vi "peak_detection.vi"(0 "Array":dbl[](array[numeric])) -> (1 "upper":dbl[](array[numeric]), 2 "upper time":dbl[](array[numeric]), 3 "lower":dbl[](array[numeric]), 4 "lower time":dbl[](array[numeric]))   [LabVIEW 2018]
panel:
  # "after interplotation"
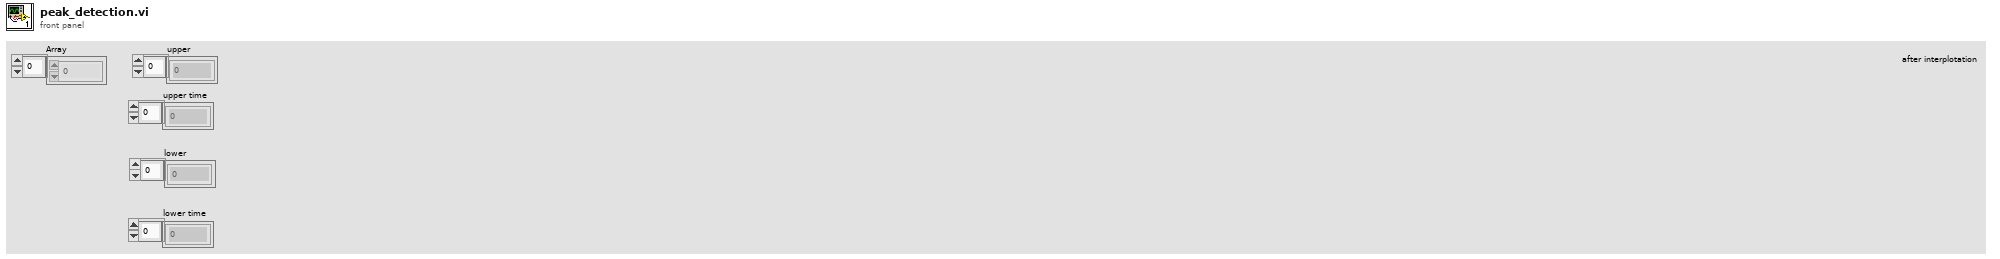
[diagram p1: front panel]
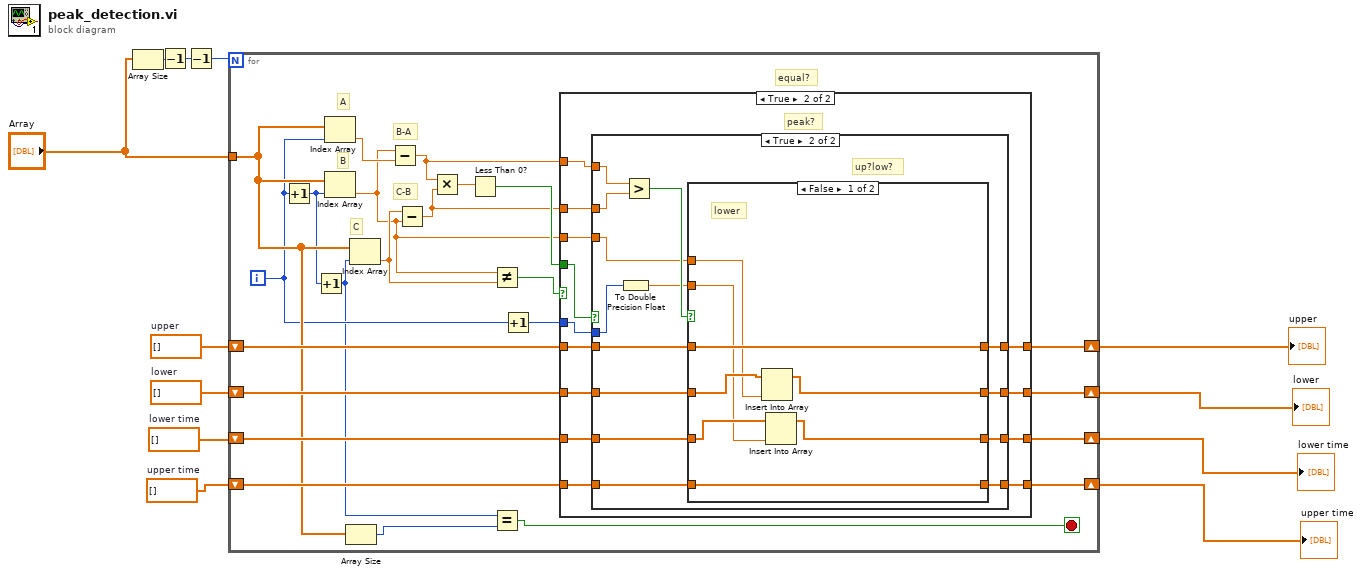
[diagram p0: block diagram]
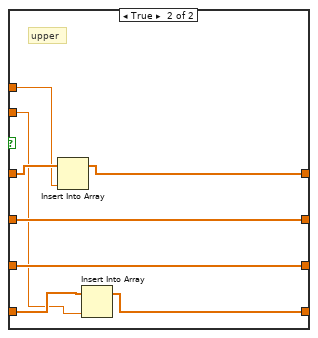
[diagram p4: hidden frame]
diagram:
  w6 = dbl[] []  # upper time
  w5 = dbl[] []  # lower time
  w4 = dbl[] []  # lower
  w3 = dbl[] []  # upper
  n1 = Array Size(array="Array") -> (size(s)=w11:i32)
  n2 = Decrement(x=w11) -> (x-1=w12:i32)
  n3 = Decrement(x=w12) -> (x-1=w1:i32)
  n4 = for {
    N: w1 -> [_]
    tunnel: "Array" -> [w25]
    shift-right: [w30] -> w7
    shift-left: w3 -> [w35]
    shift-right: [w29] -> w8
    shift-left: w4 -> [w34]
    shift-right: [w28] -> w9
    shift-left: w5 -> [w32]
    shift-right: [w27] -> w10
    shift-left: w6 -> [w31]
    i -> [w22]
    stop <- w24 stop-if-true
    # "equal?"
    # "C"
    # "B"
    # "A"
    # "C-B"
    # "B-A"
    n5 = Increment(x=w22) -> (x+1=w23:i32)
    n6 = Increment(x=w23) -> (x+1=w21:i32)
    n7 = Index Array(array=w25, index=w22) -> (element=w20:dbl)
    n8 = Index Array(array=w25, index=w23) -> (element=w13:dbl)
    n9 = Array Size(array=w25) -> (size(s)=w26:i32)
    n10 = Index Array(array=w25, index=w21) -> (element=w16:dbl)
    n11 = Subtract(x=w13, y=w20) -> (x-y=w15:dbl)
    n12 = Subtract(x=w16, y=w13) -> (x-y=w14:dbl)
    n13 = Multiply(x=w15, y=w14) -> (x*y=w19:dbl)
    n14 = Less Than 0?(x=w19) -> (x < 0?=w18:bool)
    n15 = Not Equal?(x=w13, y=w16) -> (x != y?=w17:bool)
    n16 = Equal?(x=w21, y=w26) -> (x = y?=w24:bool)
    n17 = Increment(x=w22) -> (x+1=w33:i32)
    n18 = case shown="True" w17 {
      tunnel: w35 -> [w39 w50]
      tunnel: w33 -> [_ w43]
      tunnel: w34 -> [w38 w48]
      tunnel: w32 -> [w37 w46]
      tunnel: w31 -> [w36 w44]
      tunnel: [w39 w51] -> w30
      tunnel: [w38 w49] -> w29
      tunnel: [w37 w47] -> w28
      tunnel: [w36 w45] -> w27
      tunnel: w18 -> [_ w52]
      tunnel: w15 -> [_ w42]
      tunnel: w14 -> [_ w41]
      tunnel: w13 -> [_ w40]
      frame False {
      }
      frame True {
        # "peak?"
        n19 = case shown="True" w52 {
          tunnel: [w56 w61] -> w51
          tunnel: w50 -> [w56 w62]
          tunnel: [w55 w67] -> w49
          tunnel: w48 -> [w55 w66]
          tunnel: [w54 w65] -> w47
          tunnel: w46 -> [w54 w64]
          tunnel: [w53 w59] -> w45
          tunnel: w44 -> [w53 w60]
          tunnel: w43 -> [_ w58]
          tunnel: w42 -> [_ w70]
          tunnel: w41 -> [_ w69]
          tunnel: w40 -> [_ w63]
          frame False {
          }
          frame True {
            # "up?low?"
            n20 = To Double Precision Float(number=w58) -> (double precision float=w57:dbl)
            n21 = Greater?(x=w70, y=w69) -> (0:w68:bool)
            n22 = case shown="False" w68 {
              tunnel: [w74 w86] -> w67
              tunnel: w66 -> [w76 w86]
              tunnel: [w71 w85] -> w65
              tunnel: w64 -> [w73 w85]
              tunnel: w63 -> [w75 w83]
              tunnel: w62 -> [w78 w84]
              tunnel: [w78 w82] -> w61
              tunnel: w60 -> [w77 w81]
              tunnel: [w77 w79] -> w59
              tunnel: w57 -> [w72 w80]
              frame False {
                # "lower"
                n23 = Insert Into Array(array=w76, new element=w75) -> (w74:dbl[])  [unwired: 1 in]
                n24 = Insert Into Array(array=w73, new element=w72) -> (w71:dbl[])  [unwired: 1 in]
              }
              frame True {
                # "upper"
                n25 = Insert Into Array(array=w84, new element=w83) -> (w82:dbl[])  [unwired: 1 in]
                n26 = Insert Into Array(array=w81, new element=w80) -> (w79:dbl[])  [unwired: 1 in]
              }
            }
          }
        }
      }
    }
  }
  "upper time" <- w10
  "lower time" <- w9
  "lower" <- w8
  "upper" <- w7
